vi "PFI-28000-Utils_Parse Boolean Value.vi"(0 "String":string, 11 "error in (no error)":errorcluster) -> (4 "Value":bool, 15 "error out":errorcluster)   [LabVIEW 2017, in "PFI-28000-Utils.lvlib"]
uses:
  PFI-28000-Utils.lvlib
  <vilib>/regexp/Match Regular Expression.xnode
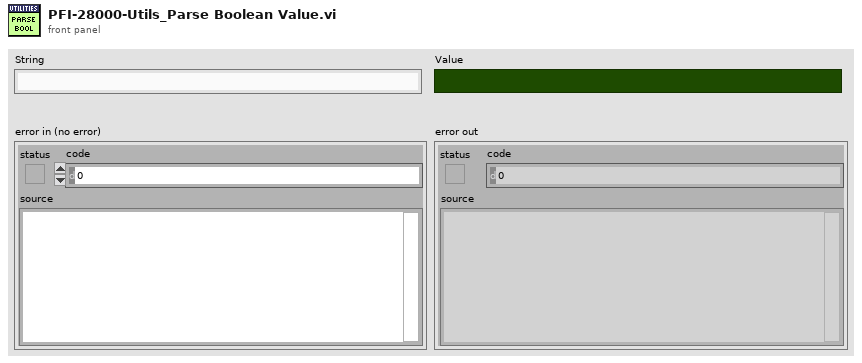
[diagram p1: front panel]
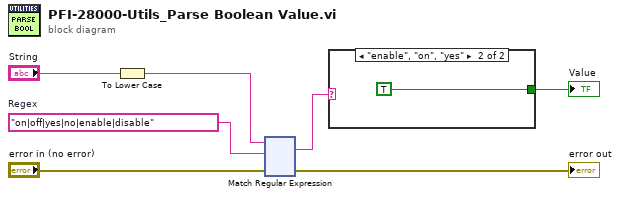
[diagram p0: block diagram]
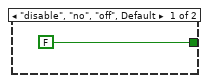
[diagram p2: hidden frame]
diagram:
  w6 = "on|off|yes|no|enable|disable"  # Regex
  n1 = To Lower Case(string="String") -> (all lower case string=w1:string)
  n2 = xnode "Match Regular Expression"("input string"=w1, "regular expression"=w6, "error in"="error in (no error)") -> ("whole match"=w5:string, "error out"=→"error out":errorcluster)  [unwired: 3 in, 3 out]
  n3 = case shown="\"enable\", \"on\", \"yes\"" w5 {
    tunnel: [FALSE TRUE] -> w4
    frame "disable", "no", "off", Default {
    }
    frame "enable", "on", "yes" {
    }
  }
  "Value" <- w4
